vi "2-Iterations Until Integer Equals Five.vi"() -> ()   [LabVIEW 2014]
panel:
  out "Random Number":dbl
  out "Random Integer":dbl
  out "Required Iterations":dbl
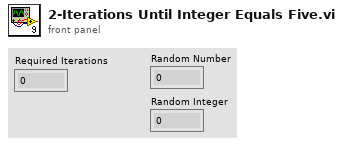
[diagram p1: front panel]
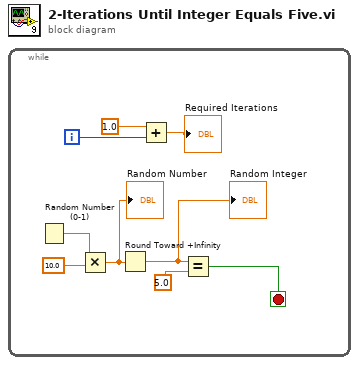
[diagram p0: block diagram]
diagram:
  n1 = while {
    i -> [w5]
    stop <- w3 stop-if-true
    n2 = Random Number (0-1)() -> (number: 0 to 1=w9:dbl)
    n3 = Multiply(x=w9, y=10.0 ("x")) -> (x*y=w2:dbl)
    "Random Number" <- w2
    n4 = Round Toward +Infinity(x=w2) -> (ceil(x): smallest int >= x=w1:dbl)
    "Random Integer" <- w1
    n5 = Add(x=1.0, y=w5) -> (x+y=→"Required Iterations":dbl)
    n6 = Equal?(x=w1, y=5.0 ("x")) -> (x = y?=w3:bool)
  }
